vi "Parse Board.vi"(0 "Board Array":T2[](array[typedef]), 5 "DT Team #":i32, 11 "error in (no error)":errorcluster) -> (4 "Parsed Board Info":T1, 15 "error out":errorcluster)   [LabVIEW 2014, in "Dragon Tamers.lvlib"]
uses:
  Dragon Tamers.lvlib
  Typedefs/Board Cell.ctl
  Typedefs/Cell Occupancy.ctl
  Typedefs/Parsed Board.ctl
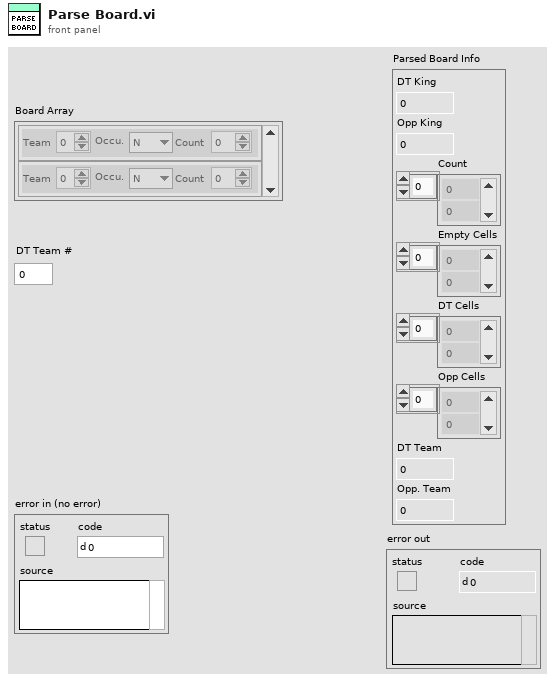
[diagram p1: front panel]
types:
  T1 = typedef "Dragon Tamers.lvlib/Parsed Board.ctl" = cluster{"DT King":i32, "Opp King":i32, "Count":i32[], "Empty Cells":i32[], "DT Cells":i32[], "Opp Cells":i32[], "DT Team":i32, "Opp. Team":i32}
  T2 = typedef "Dragon Tamers.lvlib/Board Cell.ctl" = cluster{"Team":i32, "Occu.":T3, "Count":i32}
  T3 = typedef "Dragon Tamers.lvlib/Cell Occupancy.ctl" = enum16{"N", "C", "K"}
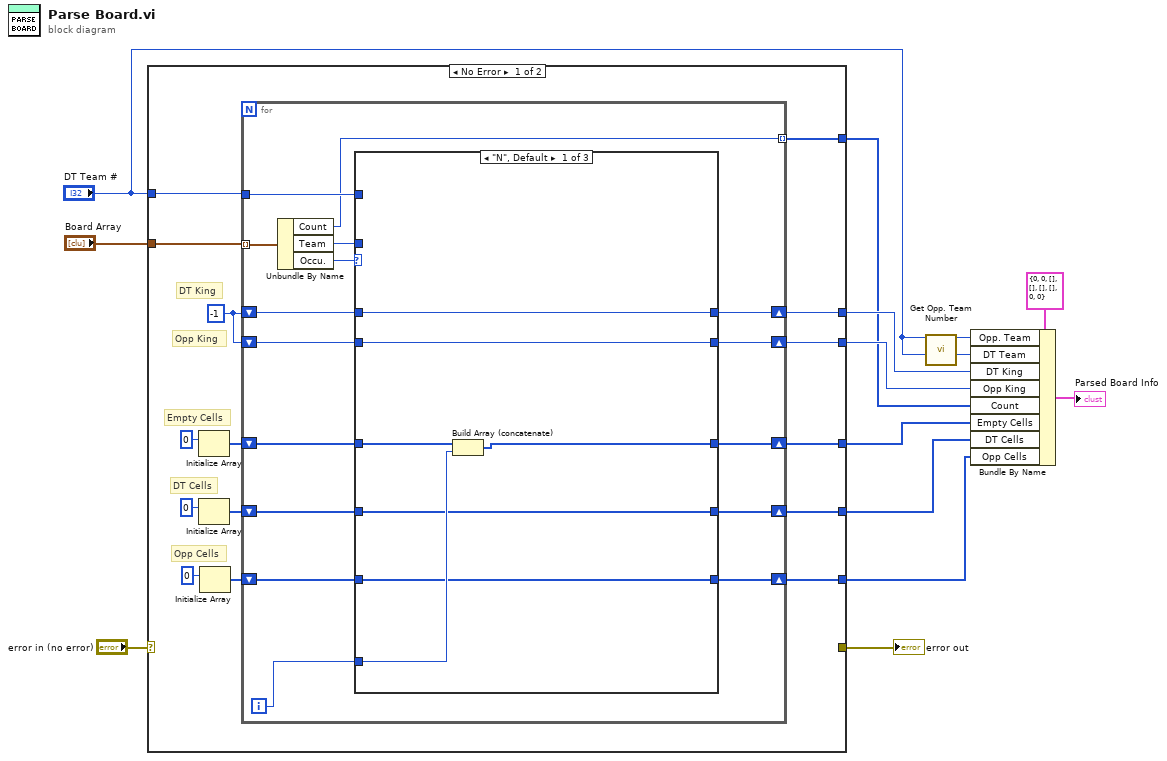
[diagram p0: block diagram]
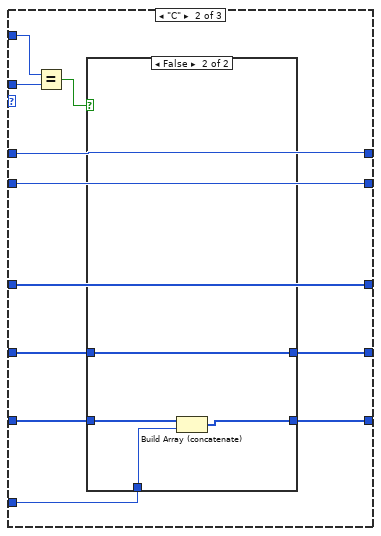
[diagram p2: hidden frame]
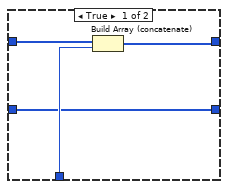
[diagram p3: hidden frame]
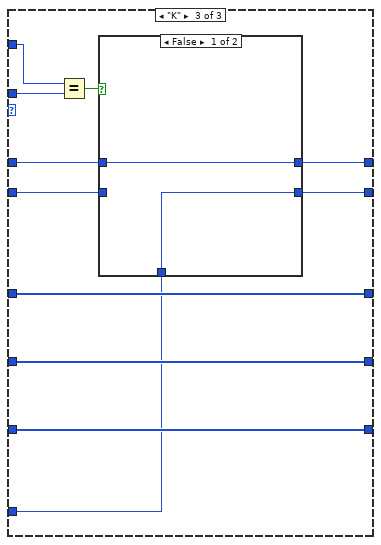
[diagram p4: hidden frame]
diagram:
  n1 = case shown="No Error" "error in (no error)" {
    selector: "error in (no error)" -> [_ w86]
    tunnel: [_ w86] -> w12
    tunnel: "Board Array" -> [w28 _]
    tunnel: "DT Team #" -> [w27 _]
    tunnel: [w19 _] -> w10
    tunnel: [w18 _] -> w9
    tunnel: [w17 _] -> w8
    tunnel: [w16 _] -> w7
    tunnel: [w15 _] -> w6
    tunnel: [w14 _] -> w5
    frame No Error {
      w20 = -1
      # "Empty Cells"
      # "Opp King"
      # "DT King"
      # "Opp Cells"
      # "DT Cells"
      n2 = Initialize Array(0) -> (w26:i32[])  [unwired: 1 in]
      n3 = Initialize Array(0) -> (w23:i32[])  [unwired: 1 in]
      n4 = Initialize Array(0) -> (w22:i32[])  [unwired: 1 in]
      n5 = for {
        tunnel: w28 -> [w44] mode=indexing
        tunnel: w27 -> [w41]
        shift-right: [w37] -> w16
        shift-left: w26 -> [w40]
        shift-right: [w34] -> w15
        shift-left: w23 -> [w39]
        shift-right: [w35] -> w14
        shift-left: w22 -> [w38]
        shift-right: [w30] -> w18
        shift-left: w20 -> [w32]
        shift-right: [w31] -> w19
        shift-left: w20 -> [w33]
        tunnel: [w29] -> w17 mode=indexing
        i -> [w42]
        n6 = Unbundle By Name(w44) -> ("Count"=w29:i32, "Team"=w36:i32, "Occu."=w43:T3)
        n7 = case shown="\"N\", Default" w43 {
          tunnel: w42 -> [w50 w57 w73]
          tunnel: w41 -> [_ w61 w78]
          tunnel: w40 -> [w51 w62 w81]
          tunnel: w39 -> [w48 w58 w80]
          tunnel: w38 -> [w47 w56 w79]
          tunnel: [w49 w62 w81] -> w37
          tunnel: w36 -> [_ w60 w77]
          tunnel: [w47 w55 w79] -> w35
          tunnel: [w48 w54 w80] -> w34
          tunnel: w33 -> [w46 w53 w75]
          tunnel: w32 -> [w45 w52 w74]
          tunnel: [w46 w53 w72] -> w31
          tunnel: [w45 w52 w71] -> w30
          frame "N", Default {
            n8 = Build Array (concatenate)(w51, w50) -> (w49:i32[])
          }
          frame "C" {
            n9 = Equal?(x=w61, y=w60) -> (x = y?=w59:bool)
            n10 = case shown="False" w59 {
              tunnel: w58 -> [w66 w67]
              tunnel: w57 -> [w65 w69]
              tunnel: w56 -> [w63 w70]
              tunnel: [w63 w68] -> w55
              tunnel: [w64 w67] -> w54
              frame True {
                n11 = Build Array (concatenate)(w66, w65) -> (w64:i32[])
              }
              frame False {
                n12 = Build Array (concatenate)(w70, w69) -> (w68:i32[])
              }
            }
          }
          frame "K" {
            n13 = Equal?(x=w78, y=w77) -> (x = y?=w76:bool)
            n14 = case shown="False" w76 {
              tunnel: w75 -> [w82 _]
              tunnel: w74 -> [_ w84]
              tunnel: w73 -> [w83 w85]
              tunnel: [w82 w85] -> w72
              tunnel: [w83 w84] -> w71
              frame False {
              }
              frame True {
              }
            }
          }
        }
      }
    }
    frame Error {
    }
  }
  "error out" <- w12
  n15 = call "Get Opp. Team Number.vi"("DT Team"="DT Team #") -> ("Opp Team"=w2:i32)  [unwired: 14 in]
  n16 = Bundle By Name(cluster=T1 {"DT King"=0, "Opp King"=0, "Count"=[], "Empty Cells"=[], "DT Cells"=[], "Opp Cells"=[], "DT Team"=0, "Opp. Team"=0} ("Parsed Board Info"), "Opp. Team"=w2, "DT Team"="DT Team #", "DT King"=w10, "Opp King"=w9, "Count"=w8, "Empty Cells"=w7, "DT Cells"=w6, "Opp Cells"=w5) -> (→"Parsed Board Info":T1)
